vi "Ref_Sts_ch_11-20.vi"(0 "Status Ch 11":refnum<vi>, 1 "Status Ch 12":refnum<vi>, 2 "Status Ch 13":refnum<vi>, 3 "Status Ch 14":refnum<vi>, 4 "Status Ch 15":refnum<vi>, 5 "Status Ch 16":refnum<vi>, 6 "Status Ch 17":refnum<vi>, 7 "Status Ch 18":refnum<vi>, 8 "Status Ch 19":refnum<vi>, 9 "Status Ch 20":refnum<vi>, 14 "Init_F":bool=TRUE) -> (18 "Status Ch 19 out":refnum<vi>, 19 "Status Ch 20 out":refnum<vi>, 20 "Status Ch 11 out":refnum<vi>, 21 "Status Ch 12 out":refnum<vi>, 22 "Status Ch 13 out":refnum<vi>, 23 "Status Ch 14 out":refnum<vi>, 24 "Status Ch 15 out":refnum<vi>, 25 "Status Ch 16 out":refnum<vi>, 26 "Status Ch 17 out":refnum<vi>, 27 "Status Ch 18 out":refnum<vi>)   [LabVIEW 2017]
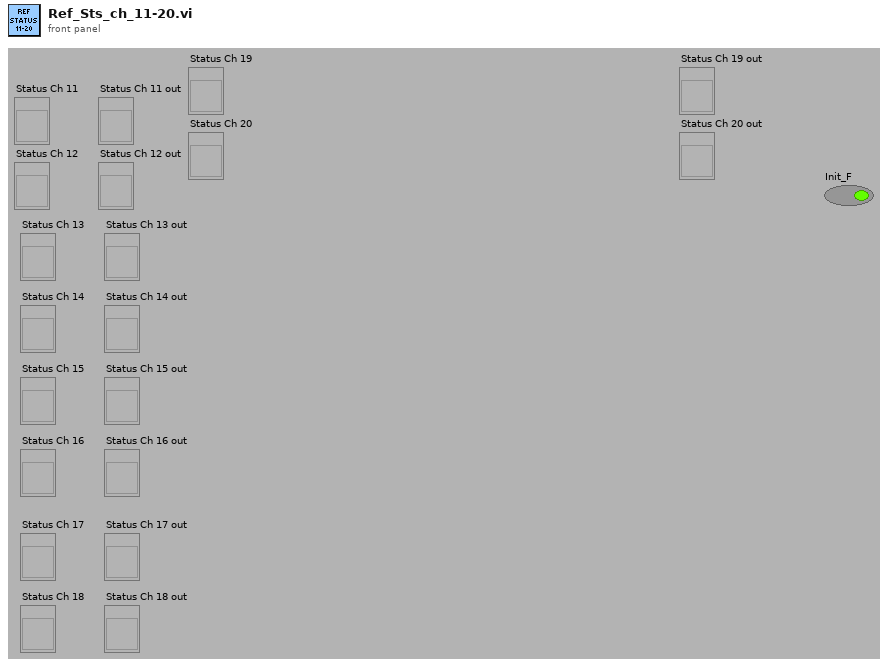
[diagram p1: front panel]
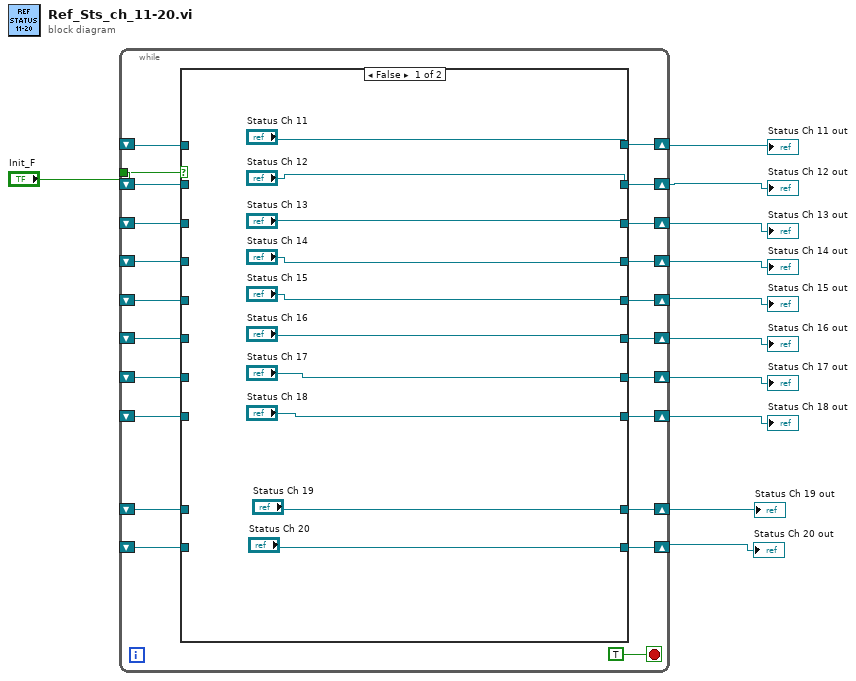
[diagram p0: block diagram]
diagram:
  n1 = while {
    shift-right: [w32] -> w3
    shift-left: _ -> [w31]
    tunnel: "Init_F" -> [w30]
    shift-right: [w29] -> w4
    shift-left: _ -> [w22]
    shift-right: [w28] -> w5
    shift-left: _ -> [w21]
    shift-right: [w27] -> w6
    shift-left: _ -> [w16]
    shift-right: [w26] -> w7
    shift-left: _ -> [w20]
    shift-right: [w25] -> w8
    shift-left: _ -> [w19]
    shift-right: [w24] -> w9
    shift-left: _ -> [w18]
    shift-right: [w23] -> w10
    shift-left: _ -> [w17]
    shift-right: [w15] -> w1
    shift-left: _ -> [w13]
    shift-right: [w14] -> w2
    shift-left: _ -> [w12]
    stop <- TRUE stop-if-true
    n2 = case shown="False" w30 {
      tunnel: ["Status Ch 11" w53] -> w32
      tunnel: w31 -> [_ w53]
      tunnel: ["Status Ch 12" w46] -> w29
      tunnel: ["Status Ch 13" w47] -> w28
      tunnel: ["Status Ch 14" w48] -> w27
      tunnel: ["Status Ch 15" w49] -> w26
      tunnel: ["Status Ch 16" w50] -> w25
      tunnel: ["Status Ch 17" w51] -> w24
      tunnel: ["Status Ch 18" w52] -> w23
      tunnel: w22 -> [_ w46]
      tunnel: w21 -> [_ w47]
      tunnel: w20 -> [_ w49]
      tunnel: w19 -> [_ w50]
      tunnel: w18 -> [_ w51]
      tunnel: w17 -> [_ w52]
      tunnel: w16 -> [_ w48]
      tunnel: ["Status Ch 19" w45] -> w15
      tunnel: ["Status Ch 20" w44] -> w14
      tunnel: w13 -> [_ w45]
      tunnel: w12 -> [_ w44]
      frame False {
      }
      frame True {
      }
    }
  }
  "Status Ch 11 out" <- w3
  "Status Ch 12 out" <- w4
  "Status Ch 13 out" <- w5
  "Status Ch 14 out" <- w6
  "Status Ch 15 out" <- w7
  "Status Ch 16 out" <- w8
  "Status Ch 17 out" <- w9
  "Status Ch 18 out" <- w10
  "Status Ch 19 out" <- w1
  "Status Ch 20 out" <- w2
